vi "tra25cc_driver.vi"(10 "user_event-status_in":refnum<user-event>, 11 "queue-commands":refnum<queue>) -> (3 "user_event-status_out":refnum<user-event>)   [LabVIEW 2018]
uses:
  <vilib>/Platform/TimedLoop/XDataNode/timing_clust.ctl
  <vilib>/Platform/TimedLoop/XDataNode/nitl_modes.ctl
  <vilib>/Platform/TimedLoop/XDataNode/wakeup.ctl
  <vilib>/platform/TimedLoop/XDataNode/XDataNode.xnode
  <vilib>/Platform/TimedLoop/XDataNode/XDNodeRunTimeDep.lvlib
panel:
  out "error out":errorcluster
  in  "error in (no error)":errorcluster
  out "command":string
  out "Y":dbl
  out "X":dbl
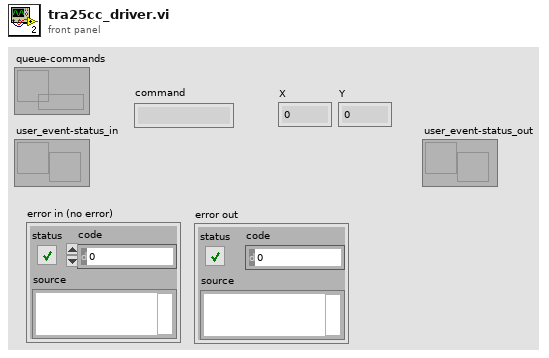
[diagram p1: front panel]
types:
  T1 = cluster{"conn_x_out":refnum<k24>, "conn_y_out":refnum<k24>, "conn_z_out":refnum<k24>}
  T2 = typedef "XDNodeRunTimeDep.lvlib/timing_clust.ctl" = cluster{"Expected End [f-1]":u64, "Actual End [f-1]":u64, "Finished Late? [f-1]":bool, "Expected End [i-1]":u64, "Actual End [i-1]":u64, "Finished Late? [i-1]":bool, "Expected Start [i]":u64, "Actual Start [i]":u64, "Expected Start [f]":u64, "Actual Start [f]":u64, "Source Name":string, "Structure Name":string, "Period":i64, "Deadline":i64, "Offset":i64, "Start":i64, "Priority":i32, "Timeout":i32, "Mode":T3, "Wakeup Reason":T4, "Error":errorcluster, "Source Type":string, "Secondary Source Type":string, "Global End Time":u64, "Global Start Time":u64, "Frame Duration":u64, "Iteration Duration":u64, "Assigned CPU":i32, "I/O Scan Engine Mode":u32}
  T3 = typedef "XDNodeRunTimeDep.lvlib/nitl_modes.ctl" = enum32{"No Change", "Process missed periods, maintain original phase", "Discard missed periods, maintain original phase", "Process missed periods, ignore original phase", "Discard missed periods, ignore original phase"}
  T4 = typedef "XDNodeRunTimeDep.lvlib/wakeup.ctl" = enum32{"Normal", "Aborted", "Asynchronous wakeup", "Timing source error", "Timed loop error", "Timeout"}
  T5 = cluster{"Enum":enum16{"standby", "domove", "dostop", "exit", "status"}, "Numeric Control":dbl, "Numeric Control":dbl, "Numeric Control":dbl}
  T6 = enum16{"standby", "domove", "dostop", "exit", "status"}
  T7 = cluster{"Numeric Control":dbl, "Numeric Control":dbl}
  T8 = cluster{"controllerState":u32, "controllerState":u32, "controllerState":u32}
  T9 = cluster{"controllerState":u32, "controllerState":u32, "controllerState":u32, "pos_x":dbl, "pos_y":dbl, "pos_z":dbl}
  T10 = cluster{enum16{"standby", "domove", "dostop", "exit", "status"}, dbl, dbl, dbl}
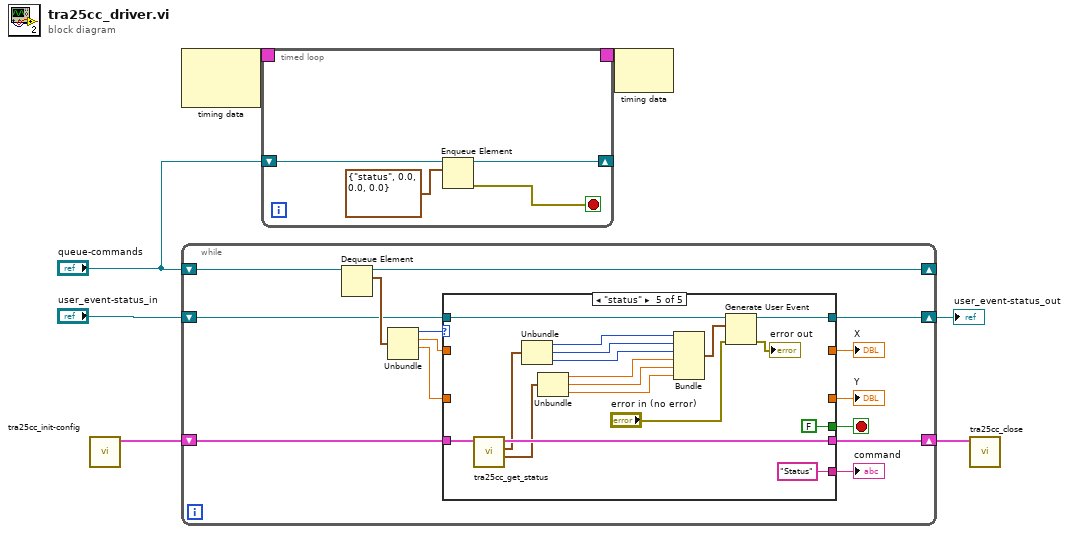
[diagram p0: block diagram]
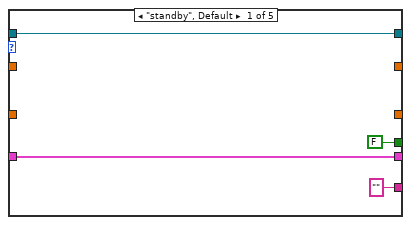
[diagram p2: hidden frame]
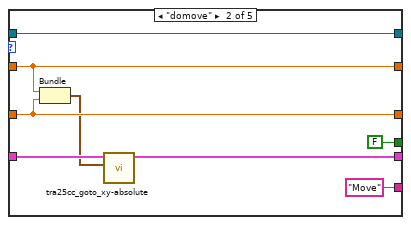
[diagram p3: hidden frame]
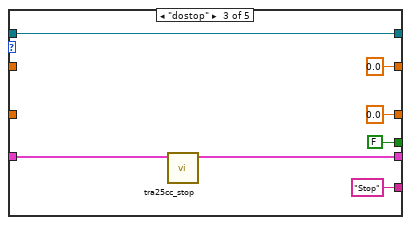
[diagram p4: hidden frame]
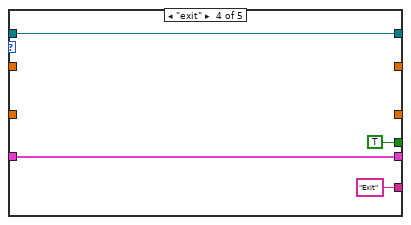
[diagram p5: hidden frame]
diagram:
  n1 = call "tra25cc_init-config.vi"() -> ("conn_xyz_out"=w2:T1)  [unwired: 11 in]
  n2 = node-c288() -> (w5:T2)  [unwired: 2 in]
  n3 = while {
    shift-right: [w11] -> w6
    shift-left: "user_event-status_in" -> [w12]
    shift-right: [w10] -> _
    shift-left: "queue-commands" -> [w14]
    shift-right: [w8] -> w1
    shift-left: w2 -> [w9]
    stop <- w13 stop-if-true
    n4 = Dequeue Element(queue=w14) -> (queue out=w10:refnum<queue>, element=w18:T5)  [unwired: 2 in, 2 out]
    n5 = Unbundle(w18) -> ("Enum"=w17:T6, "Numeric Control"=w16:dbl, "Numeric Control"=w15:dbl)  [unwired: 1 out]
    n6 = case shown="\"status\"" w17 {
      tunnel: ["" ("command") "Move" ("command") "Stop" ("command") "Exit" ("command") "Status" ("command")] -> w21
      tunnel: [_ w28 0.0 _ _] -> w20
      tunnel: [_ w27 0.0 _ _] -> w19
      tunnel: [FALSE FALSE FALSE TRUE FALSE] -> w13
      tunnel: w16 -> [_ w28 _ _ _]
      tunnel: w15 -> [_ w27 _ _ _]
      tunnel: w12 -> [w23 w31 w36 w42 w59]
      tunnel: [w23 w31 w36 w42 w58] -> w11
      tunnel: w9 -> [w22 w30 w35 w41 w54]
      tunnel: [w22 w29 w34 w41 w53] -> w8
      frame "standby", Default {
      }
      frame "domove" {
        n7 = Bundle("Numeric Control"=w28, "Numeric Control"=w27) -> (w26:T7)  [unwired: 1 in]
        n8 = call "tra25cc_goto_xy-absolute.vi"("xy_val_mm"=w26, "conn_xyz_in"=w30) -> ("conn_xyz_out"=w29:T1)  [unwired: 8 in, 1 out]
      }
      frame "dostop" {
        n9 = call "tra25cc_stop.vi"("conn_xyz_in"=w35) -> ("conn_xyz_out"=w34:T1)  [unwired: 9 in, 1 out]
      }
      frame "exit" {
      }
      frame "status" {
        n10 = call "tra25cc_get_status.vi"("conn_xyz_in"=w54) -> ("position_xyz"=w51:cluster{"pos_x":dbl, "pos_y":dbl, "pos_z":dbl}, "state_xyz"=w52:T8, "conn_xyz_out"=w53:T1)  [unwired: 6 in, 2 out]
        n11 = Unbundle(w52) -> ("controllerState"=w50:u32, "controllerState"=w49:u32, "controllerState"=w48:u32)
        n12 = Unbundle(w51) -> ("pos_x"=w47:dbl, "pos_y"=w46:dbl, "pos_z"=w45:dbl)
        n13 = Bundle("controllerState"=w50, "controllerState"=w49, "controllerState"=w48, "pos_x"=w47, "pos_y"=w46, "pos_z"=w45) -> (w57:T9)  [unwired: 1 in]
        n14 = Generate User Event(user event=w59, event data cluster=w57, error in="error in (no error)") -> (user event out=w58:refnum<user-event>, error out=→"error out":errorcluster)  [unwired: 1 in]
      }
    }
    "command" <- w21
    "X" <- w20
    "Y" <- w19
  }
  "user_event-status_out" <- w6
  n15 = timed-loop {
    timing: w5 -> [_]
    timing-out: [_] -> w4
    shift-right: [w62] -> _
    shift-left: "queue-commands" -> [w64]
    stop <- w63 stop-if-true
    n16 = Enqueue Element(queue=w64, element=T10 {enum."status", 0.0, 0.0, 0.0}) -> (queue out=w62:refnum<queue>, error out=w63:errorcluster)  [unwired: 2 in, 1 out]
  }
  n17 = node-c288(w4) -> ()  [unwired: 1 out]
  n18 = call "tra25cc_close.vi"("conn_xyz_in"=w1) -> ()  [unwired: 10 in, 1 out]
